vi "Set_Parameter_Instrument (Json).vi"(8 "error in (no error)":errorcluster caption="entrée d'erreur (pas d'erreur)", 10 "Parameter (Json)":string, 11 "Flash_Jlink en entrée":refnum<class "Flash_AVRDUDE.lvclass">) -> (0 "error out":errorcluster caption="sortie d'erreur", 3 "Flash_Jlink en sortie":refnum<class "Flash_AVRDUDE.lvclass">)   [LabVIEW 2020, in "Library Test.lvlib" / "Flash_AVRDUDE.lvclass"]
uses:
  Flash_AVRDUDE.lvclass
  C:/Users/ngarcin/OneDrive - Altyor/Standard TB/Class/Test/Test (Default)/Test (Default).lvclass
  Commun VI/TypeDef/Commande Test/Commande Parameter Flash_.AVRDUDEctl.ctl
  Flash_AVRDUDE.lvclass/Flash_AVRDUDE.ctl
  JSON API/JSON Value/Set from JSON string.vi
  Test_Without_Instr/Test_Without_Inst.lvclass
  JSON API/JSON Value/JSON Value.lvclass
  JSON API/Variant JSON/Variant JSON.lvlib
  JSON API/Get Polymorphic/JSON GetSet.lvlib
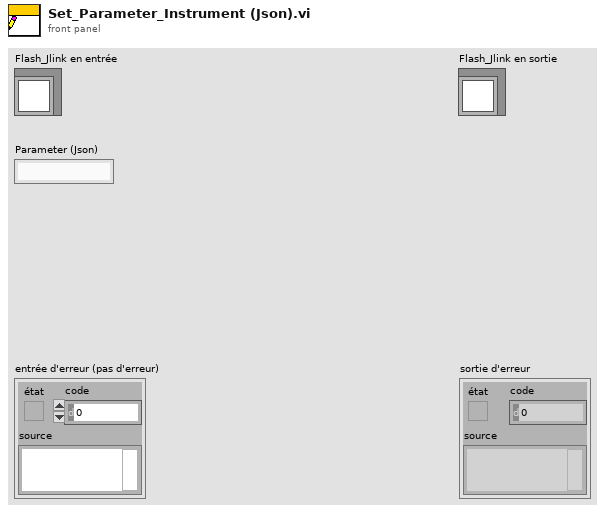
[diagram p1: front panel]
types:
  T1 = typedef "Commande Parameter Flash_.AVRDUDEctl.ctl" = cluster{"Path FW ":path, "Working Directory":path, "Device":string, "Frequency":string}
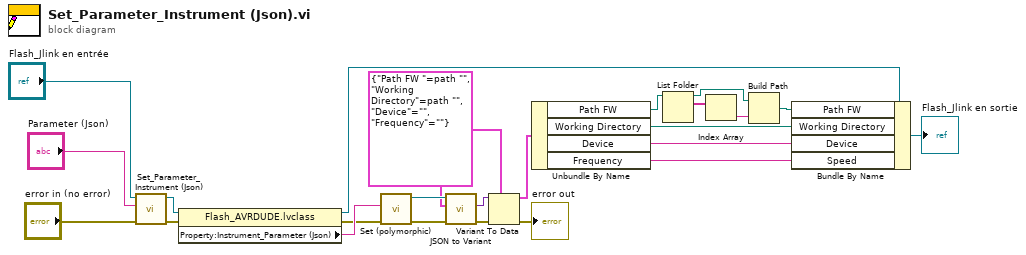
[diagram p0: block diagram]
diagram:
  w14 = T1 {"Path FW "=path "", "Working Directory"=path "", "Device"="", "Frequency"=""}
  n1 = call-parent "Set_Parameter_Instrument (Json).vi"("error in (no error)"="error in (no error)", "Parameter (Json)"="Parameter (Json)", "Test (Default) en entrée"="Flash_Jlink en entrée") -> ("error out"=w13:errorcluster, "Test (Default) en sortie"=w16:refnum<class "Flash_AVRDUDE.lvclass">)  [unwired: 7 in]
  n2 = property class="Flash_AVRDUDE.lvclass"(reference=w16, error in=w13) -> (reference out=w12:refnum<class "Flash_AVRDUDE.lvclass">, error out=w10:errorcluster, "Property:Instrument_Parameter (Json)"=w15:string)
  n3 = call-poly "Set (polymorphic).vi"("error in (no error)"=w10, "JSON stream"=w15) -> ("error out"=w18:errorcluster, "JSON Value out"=w20:refnum<class "JSON Value.lvclass">)  [unwired: 7 in, 1 out]
  n4 = call "JSON to Variant.vi"("error in (no error)"=w18, "Variant (Data Type)"=w14, "JSON Value"=w20) -> ("error out"=w19:errorcluster, "Variant out"=w17:variant)  [unwired: 7 in]
  n5 = Variant To Data(error in=w19, type=w14, Variant=w17) -> (data=w11:T1, error out=→"error out":errorcluster)
  n6 = Unbundle By Name(w11) -> ("Path FW"=w2:path, "Working Directory"=w8:path, "Device"=w7:string, "Frequency"=w6:string)
  n7 = List Folder(path=w2) -> (path out=w3:path, filenames=w5:string[])  [unwired: 3 in, 2 out]
  n8 = Index Array(array=w5) -> (element=w4:string)  [unwired: 1 in]
  n9 = Build Path(base path=w3, name or relative path=w4) -> (appended path=w1:path)
  n10 = Bundle By Name(cluster=w12, "Path FW"=w1, "Working Directory"=w8, "Device"=w7, "Speed"=w6) -> (→"Flash_Jlink en sortie":refnum<class "Flash_AVRDUDE.lvclass">)
